vi "Extract Default Icon Data.vi"(6 "Color Icon":T5, 7 "BW Icon":T5, 8 "error in (no error)":errorcluster, 9 "New VI template? (F)":bool, 11 "Body text":T7={"Line 1 text"="", "Line 2 text"="", "Line 3 text"="", "Line 4 text"="", "Line 1 color"=0, "Line 2 color"=0, "Line 3 color"=0, "Line 4 color"=0, "Body Text Spec"={"DNL_Font"="Small Fonts", "Alignment"=1, "Size"=8}, "Center text vertically"=TRUE, "Capitalize Text"=TRUE} {"Body Text Spec"."Alignment" items=["left", "center", "right"]}) -> (0 "error out":errorcluster, 2 "VI Icon Data out":T1={"Text Visible?"=TRUE, "Text Opacity"=100, "Templ Visible?"=TRUE, "Templ Opacity"=100, "Relative Path from 1 to 2"=path "", "Image"=bytes[0], "All User Layers"=[refnum], "Body Text"={"Line 1 text"="", "Line 2 text"="", "Line 3 text"="", "Line 4 text"="", "Line 1 color"=0, "Line 2 color"=0, "Line 3 color"=0, "Line 4 color"=0, "Body Text Spec"={"Font"="Small Fonts", "Alignment"=1, "Size"=9}, "Center text vertically"=TRUE, "Capitalize Text"=TRUE}} {"Body Text"."Body Text Spec"."Alignment" items=["left", "center", "right"]}, 3 "Default Icon Template data":T6={"LayerIcon"=bytes[0], "LayerName"="", "Opacity"=100, "Visibility?"=TRUE} {"Opacity" scale=0.0..100.0})   [LabVIEW 2021, in "LabVIEW Icon API.lvlib"]
doc: "Extract the default Icon Data."
uses:
  LabVIEW Icon API.lvlib
  Controls/Font.ctl
  Controls/Alignment.ctl
  <vilib>/picture/picture.llb/imagedata.ctl
  Controls/Layer.ctl
  Controls/LabVIEW Icon Stored Information.ctl
  Classes/Layer/Layer.lvclass
  Controls/BodyText.ctl
  lv_icon.lvlib
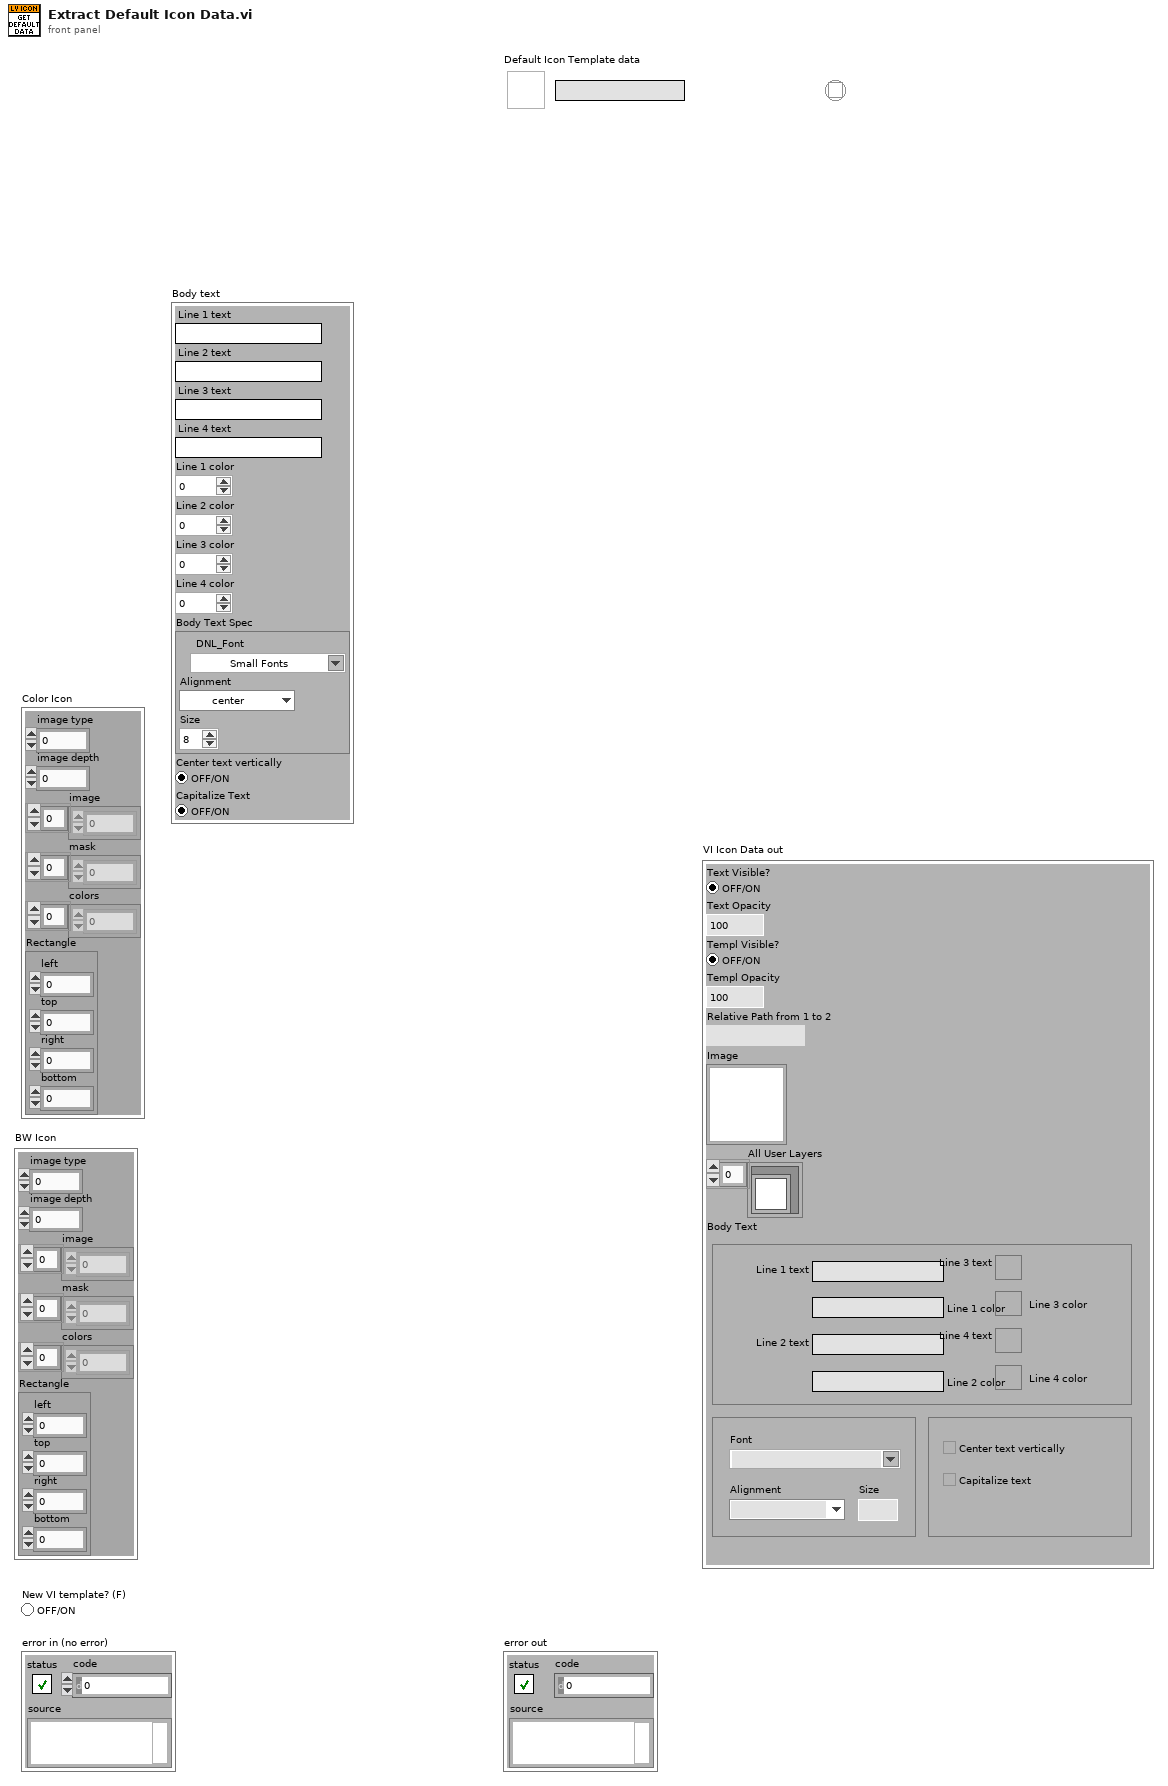
[diagram p1: front panel]
types:
  T1 = typedef "LabVIEW Icon Stored Information.ctl" = cluster{"Text Visible?":bool, "Text Opacity":u8, "Templ Visible?":bool, "Templ Opacity":u8, "Relative Path from 1 to 2":path, "Image":picture, "All User Layers":refnum<class "Layer.lvclass">[], "Body Text":T2}
  T2 = typedef "BodyText.ctl" = cluster{"Line 1 text":string, "Line 2 text":string, "Line 3 text":string, "Line 4 text":string, "Line 1 color":u32, "Line 2 color":u32, "Line 3 color":u32, "Line 4 color":u32, "Body Text Spec":cluster{"Font":T3, "Alignment":T4, "Size":u8}, "Center text vertically":bool, "Capitalize Text":bool}
  T3 = typedef "Font.ctl" = string
  T4 = typedef "Alignment.ctl" = u16
  T5 = typedef "imagedata.ctl" = cluster{"image type":i32, "image depth":i32, "image":u8[], "mask":u8[], "colors":u32[], "Rectangle":cluster{"left":i16, "top":i16, "right":i16, "bottom":i16}}
  T6 = typedef "Layer.ctl" = cluster{"LayerIcon":picture, "LayerName":string, "Opacity":u8, "Visibility?":bool}
  T7 = cluster{"Line 1 text":string, "Line 2 text":string, "Line 3 text":string, "Line 4 text":string, "Line 1 color":u32, "Line 2 color":u32, "Line 3 color":u32, "Line 4 color":u32, "Body Text Spec":cluster{"DNL_Font":T3, "Alignment":T4, "Size":u8}, "Center text vertically":bool, "Capitalize Text":bool}
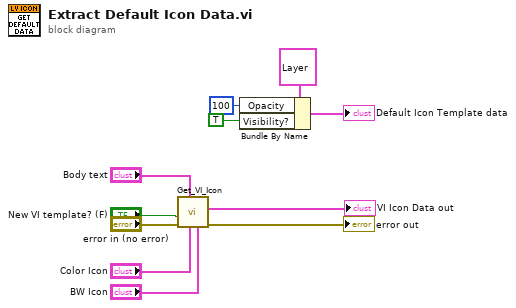
[diagram p0: block diagram]
diagram:
  n1 = call "Get_VI_Icon.vi"("BW Icon"="BW Icon", "Color Icon"="Color Icon", "Body Text"="Body text", "error in (no error)"="error in (no error)", "New VI template? (F)"="New VI template? (F)") -> ("error out"=→"error out":errorcluster, "VI Icon Data out"=→"VI Icon Data out":T1)  [unwired: 5 in]
  n2 = Bundle By Name(cluster=T6 {"LayerIcon"=bytes[0], "LayerName"="", "Opacity"=0, "Visibility?"=FALSE} ("Data"), "Opacity"=u8 100, "Visibility?"=TRUE) -> (→"Default Icon Template data":T6)
